vi "Gyro PID Back Dis.vi"(6 "Target angle":sgl, 7 "Threshold to stop":i32=1200, 8 "Threshold to slow":i32=1000, 9 "Min. speed":i32=40, 10 "Max. speed":i32=80, 11 "EV3 in":T1) -> (3 "EV3 out":T1)   [LabVIEW 2015]
uses:
  <vilib>/NXT/Block Support/NXT_OutputPort.ctl
  <vilib>/NXT/LegoClasses/BrickReference/BrickReference.lvclass
  <vilib>/NXT/Subs/LVHSConnector.ctl
  <vilib>/NXT/NXTIO Xnodes/NXTIOXNode/NXTIO.xnode
  <vilib>/NXT/Dual Mode Library/Motors/Rotation.vi
  <vilib>/NXT/Dual Mode Library/Waits/Wait_Num.vi
  <vilib>/NXT/NXTIO Xnodes/NXTIONodeSubVIs/LEGOResetMotors.vi
  <vilib>/NXT/NXTIO Xnodes/NXTIONodeSubVIs/NXTMotorSteeringOn.vi
  <vilib>/NXT/NXTIO Xnodes/NXTIONodeSubVIs/NXTStopMotors.vi
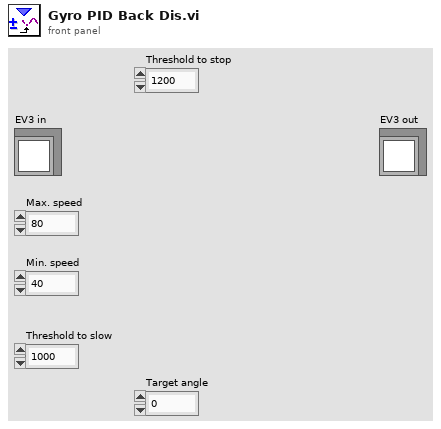
[diagram p1: front panel]
types:
  T1 = typedef "LVHSConnector.ctl" = refnum<class "BrickReference.lvclass">
  T2 = typedef "NXT_OutputPort.ctl" = u8
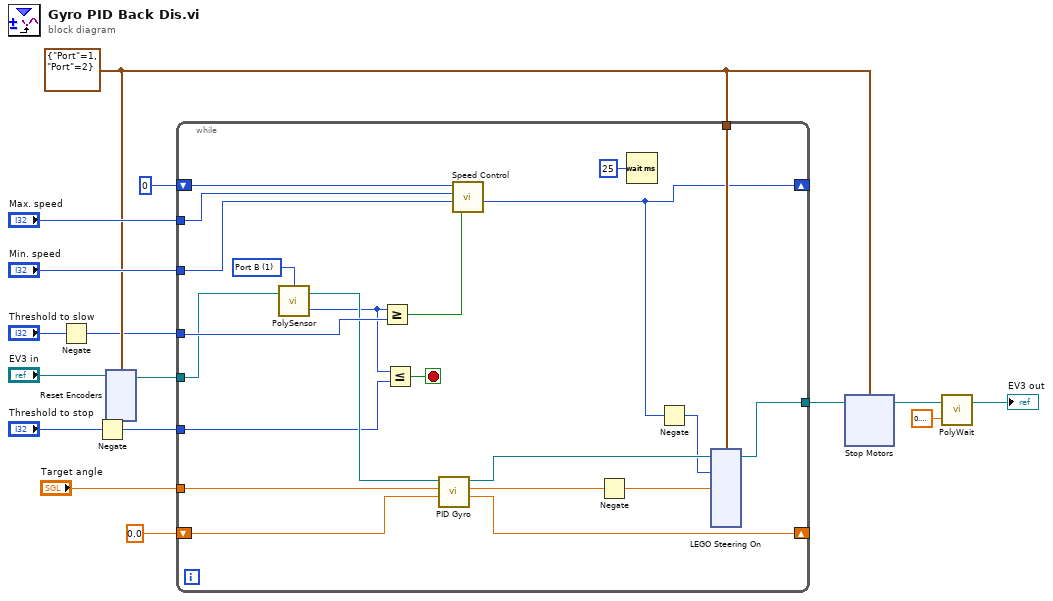
[diagram p0: block diagram]
diagram:
  w6 = cluster{"Port":T2, "Port":T2} {"Port"=1, "Port"=2} ("Motor")
  n1 = Negate(x="Threshold to slow") -> (-x=w2:i32)
  n2 = Negate(x="Threshold to stop") -> (-x=w1:i32)
  n3 = xnode "Reset Encoders"("Motors"=w6, "NXT/EV3"="EV3 in") -> ("NXT/EV3"=w12:T1)
  n4 = while {
    tunnel: w12 -> [w27]
    shift-right: [w38] -> _
    shift-left: sgl 0.0 -> [w21]
    tunnel: "Target angle" -> [w37]
    tunnel: [w34] -> w8
    tunnel: w6 -> [w36]
    shift-right: [w20] -> _
    shift-left: 0 -> [w31]
    tunnel: "Min. speed" -> [w28]
    tunnel: "Max. speed" -> [w30]
    tunnel: w2 -> [w29]
    tunnel: w1 -> [w19]
    stop <- w24 stop-if-true
    w35 = T2 1 items=["Port A", "Port B", "Port C", "Port D"] ("Port (Port A)")
    n5 = call-poly <vilib>:"PolySensor.vi"("NXT/EV3"=w27, "Port (Port A)"=w35) -> ("Angle of Rotation"=w23:i32, "NXT/EV3"=w26:T1)  [unwired: 1 in]
    n6 = Greater Or Equal?(x=w23, y=w29) -> (x >= y?=w25:bool)
    n7 = Less Or Equal?(x=w23, y=w19) -> (x <= y?=w24:bool)
    n8 = call "PID Gyro.vi"("Previous integral"=w21, "Target angle"=w37, "EV3 in"=w26) -> ("New integral"=w38:sgl, "Total error"=w32:sgl, "EV3 out"=w22:T1)  [unwired: 6 in]
    n9 = call "Speed Control.vi"("Speed Up or Down?"=w25, "Min. speed"=w28, "Max. speed"=w30, "Ini. speed"=w31) -> ("Speed out"=w20:i32)  [unwired: 7 in]
    n10 = Negate(x=w32) -> (-x=w17:sgl)
    n11 = Wait (ms)(milliseconds to wait=u32 25) -> ()  [unwired: 1 out]
    n12 = Negate(x=w20) -> (-x=w18:i32)
    n13 = xnode "LEGO Steering On"("Steering 1"=w17, "Power 1"=w18, "Motors"=w36, "NXT/EV3"=w22) -> ("NXT/EV3"=w34:T1)
  }
  n14 = xnode "Stop Motors"("Motors"=w6, "NXT/EV3"=w8) -> ("NXT/EV3"=w7:T1)
  n15 = call-poly <vilib>:"PolyWait.vi"("Time (1 sec)"=sgl 0.2, "NXT/EV3"=w7) -> ("NXT/EV3"=→"EV3 out":T1)  [unwired: 2 in]
